vi "shift regiter.vi"() -> ()   [LabVIEW 2012]
panel:
  out "Numeric":i32
  in  "stop":bool
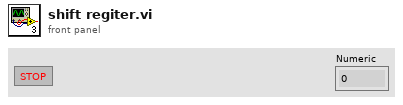
[diagram p1: front panel]
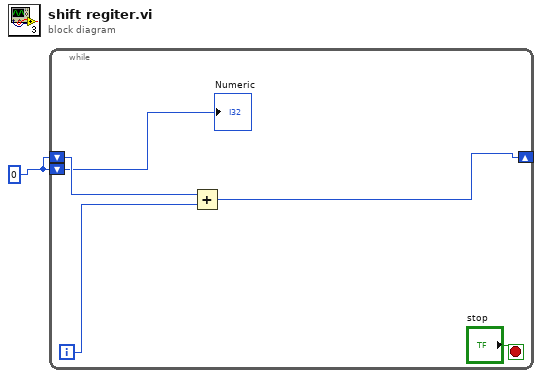
[diagram p0: block diagram]
diagram:
  w1 = 0
  n1 = while {
    shift-right: [w3] -> _
    shift-left: w1 -> [w4]
    shift-left: w1 -> [w2]
    i -> [w5]
    stop <- "stop" stop-if-true
    n2 = Add(x=w4, y=w5) -> (x+y=w3:i32)
    "Numeric" <- w2
  }
